vi "Itertools_Product.vi"(8 "Error In":errorcluster, 11 "Array List (in)":string[][](array[string])) -> (0 "Error Out":errorcluster, 2 "Product Indicies Array (Out)":i32[][](array[numeric]), 3 "Product Flattened String-Array (Out)":string[](array[string]))   [LabVIEW 2017]
doc: "ITERTOOLS - Cartesian Product:\n\nThis VI provides a fast way to calculate the cartesian product of a string array or any arbitrary data-type.\n\nThe input is a string array, where each row is a vector. \nEmpty array-elements will be filtered out.\nYou can use the \"index-table\" from the output to implement your own function for handling specific data-type."
uses:
  <userlib>/_OpenG.lib/array/array.llb/Filter 1D Array with Scalar (String)__ogtk.vi
panel:
  out "size(s) 2":i32
  out "size(s)":i32
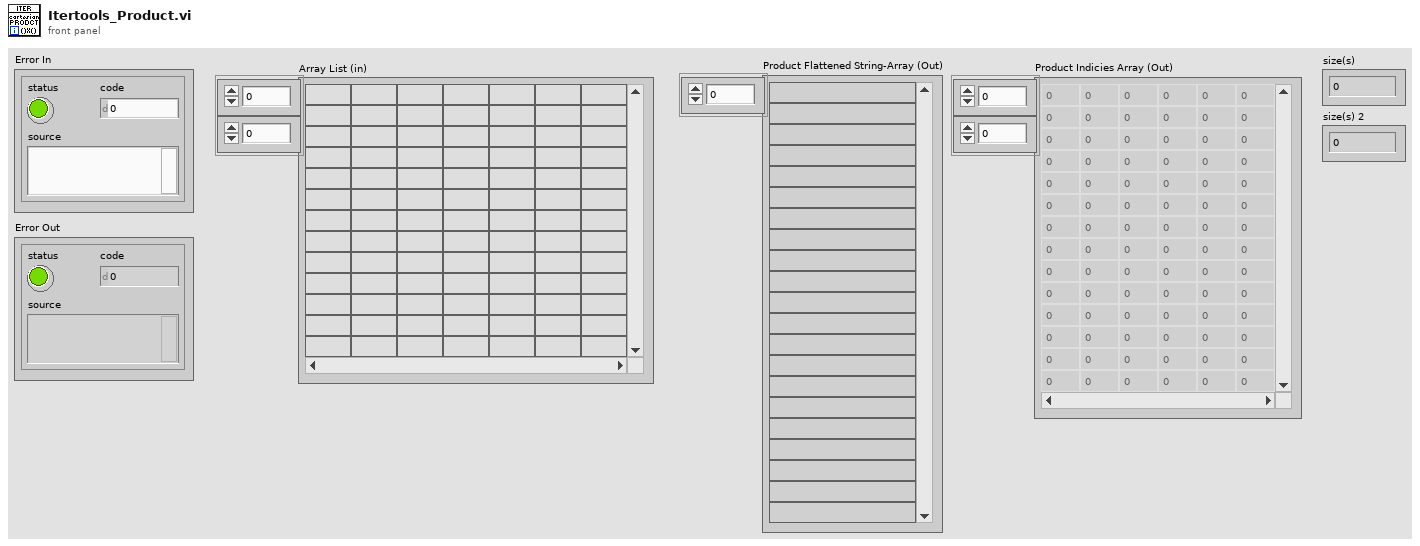
[diagram p1: front panel]
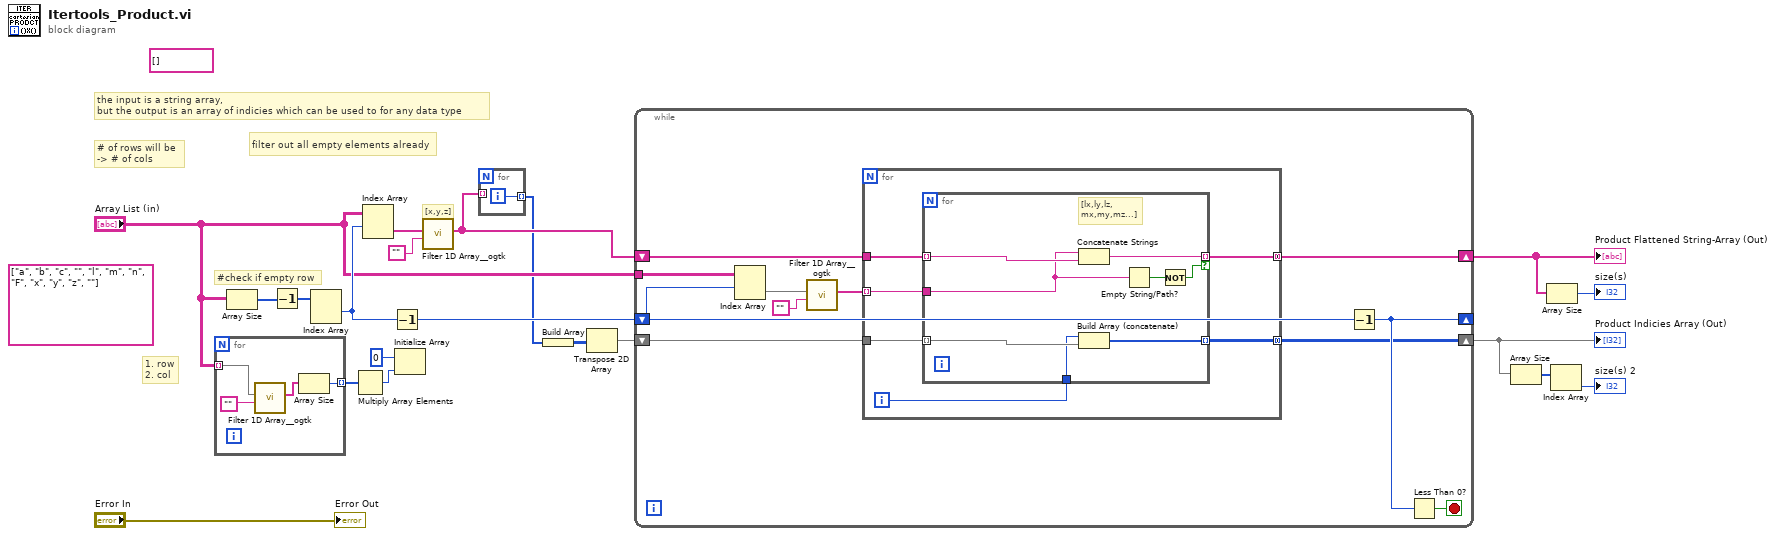
[diagram p0: block diagram]
diagram:
  (unwired) string[][] [["a", "b", "c", ""], ["l", "m", "n", "F"], ["x", "y", "z", ""]] ("Array String")
  (unwired) string[] [] ("Array String")
  # "the input is a string array,\nbut the output is an array of indicies which can be used to for any data type"
  # "#check if empty row"
  # "filter out all empty elements already"
  # "1. row\n2. col"
  # "# of rows will be\n-> # of cols"
  # "[x,y,z]"
  n1 = for {
    tunnel: "Array List (in)" -> [w22] mode=indexing
    tunnel: [w24] -> w10 mode=indexing
    n2 = call-poly <userlib>:"Filter 1D Array__ogtk.vi"("items to filter"="", "array"=w22) -> ("filtered array"=w21:string[])  [unwired: 4 in, 1 out]
    n3 = Array Size(array=w21) -> (size(s)=w24:i32)
  }
  n4 = Array Size(array="Array List (in)") -> (size(s)=w15:i32[])
  n5 = Decrement(x=w15) -> (x-1=w20:i32[])
  n6 = Index Array(array=w20) -> (element #1=w14:i32)  [unwired: 2 in, 1 out]
  n7 = Multiply Array Elements(1:w10) -> (0:w9:i32)
  n8 = Index Array(array="Array List (in)", index (row)=w14) -> (element=w12:string[])  [unwired: 1 in]
  n9 = Decrement(x=w14) -> (x-1=w17:i32)
  n10 = Initialize Array(0 ("index"), w9) -> ()  [unwired: 1 out]
  n11 = call-poly <userlib>:"Filter 1D Array__ogtk.vi"("items to filter"="", "array"=w12) -> ("filtered array"=w8:string[])  [unwired: 4 in, 1 out]
  n12 = for {
    tunnel: w8 -> [_] mode=indexing
    tunnel: [w25] -> w7 mode=indexing
    i -> [w25]
  }
  n13 = Build Array(w7) -> (w5:i32[][])
  n14 = Transpose 2D Array(2D array=w5) -> (transposed array=w6:i32[][])
  n15 = while {
    tunnel: "Array List (in)" -> [w36]
    shift-right: [w33] -> _
    shift-left: w17 -> [w31]
    shift-right: [w32] -> w19
    shift-left: w8 -> [w35]
    shift-right: [w26] -> w4
    shift-left: w6 -> [w27]
    stop <- w34 stop-if-true
    n16 = Index Array(array=w36, index (row)=w31) -> (element=w29:string[])  [unwired: 1 in]
    n17 = call-poly <userlib>:"Filter 1D Array__ogtk.vi"("items to filter"="", "array"=w29) -> ("filtered array"=w28:string[])  [unwired: 4 in, 1 out]
    n18 = for {
      tunnel: w35 -> [w42]
      tunnel: [w41] -> w32 mode=concatenating
      tunnel: w28 -> [w40] mode=indexing
      tunnel: w27 -> [w37]
      tunnel: [w39] -> w26 mode=concatenating
      i -> [w38]
      n19 = for {
        tunnel: w42 -> [w50] mode=indexing
        tunnel: [w49] -> w41 mode=indexing if=w45
        tunnel: w40 -> [w46]
        tunnel: [w48] -> w39 mode=indexing
        tunnel: w37 -> [w44] mode=indexing
        tunnel: w38 -> [w43]
        # "[lx,ly,lz,\nmx,my,mz...]"
        n20 = Concatenate Strings(w46, w50) -> (w49:string)
        n21 = Build Array (concatenate)(w43, w44) -> (w48:i32[])
        n22 = Empty String/Path?(string/path=w46) -> (empty?=w47:bool)
        n23 = Not(x=w47) -> (.not. x?=w45:bool)
      }
    }
    n24 = Decrement(x=w31) -> (x-1=w33:i32)
    n25 = Less Than 0?(x=w33) -> (x < 0?=w34:bool)
  }
  "Product Flattened String-Array (Out)" <- w19
  "Product Indicies Array (Out)" <- w4
  n26 = Array Size(array=w4) -> (size(s)=w3:i32[])
  n27 = Array Size(array=w19) -> (size(s)=→"size(s)":i32)
  n28 = Index Array(array=w3) -> (element=→"size(s) 2":i32)  [unwired: 1 in]
  "Error Out" <- "Error In"
